vi "SPI Flash Init.vi"(7 "pConfig":T1, 9 "ClockSpeed":i32, 10 "SPIIndex":i32, 11 "DevHandle":i32) -> (3 "function return":i32, 5 "pConfig out":T1)   [LabVIEW 2010, in "usb2spi.lvlib"]
doc: "int WINAPI SPI_FlashInit(int DevHandle,int SPIIndex,int ClockSpeed, PSPI_FLASH_CONFIG pConfig);"
uses:
  usb2spi.lvlib
  USB2XXX/trunk/USB2XXX/USB2XXX/vs2010/Release/USB2XXX.dll
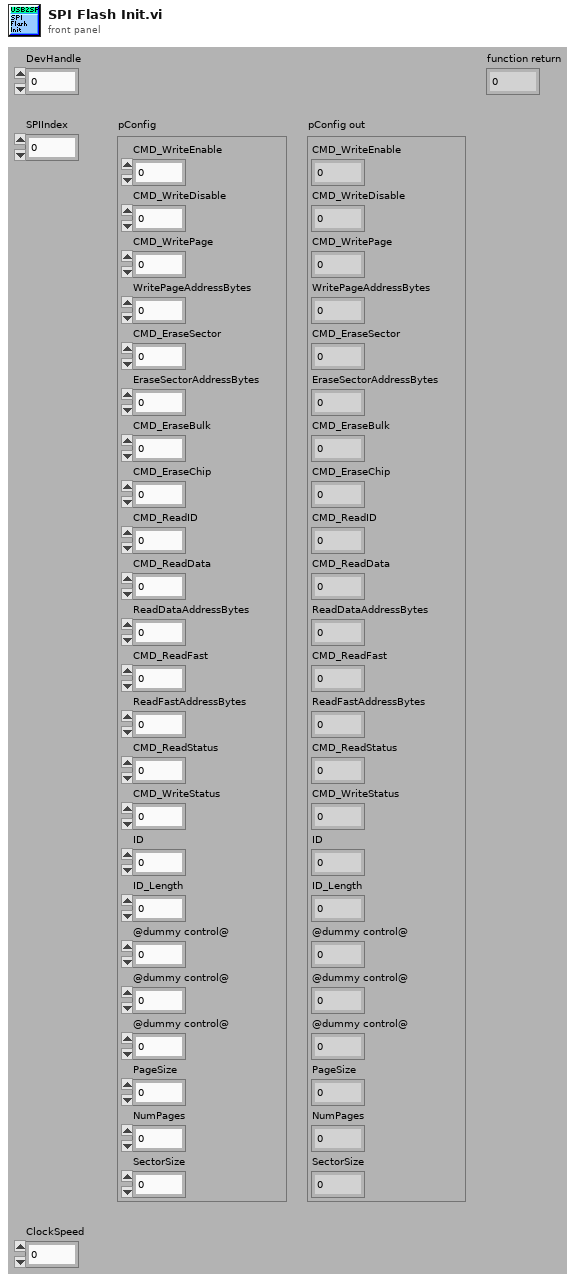
[diagram p1: front panel]
types:
  T1 = cluster{"CMD_WriteEnable":u8, "CMD_WriteDisable":u8, "CMD_WritePage":u8, "WritePageAddressBytes":u8, "CMD_EraseSector":u8, "EraseSectorAddressBytes":u8, "CMD_EraseBulk":u8, "CMD_EraseChip":u8, "CMD_ReadID":u8, "CMD_ReadData":u8, "ReadDataAddressBytes":u8, "CMD_ReadFast":u8, "ReadFastAddressBytes":u8, "CMD_ReadStatus":u8, "CMD_WriteStatus":u8, "ID":u8, "ID_Length":u8, "@dummy control@":i8, "@dummy control@":i8, "@dummy control@":i8, "PageSize":i32, "NumPages":i32, "SectorSize":i32}
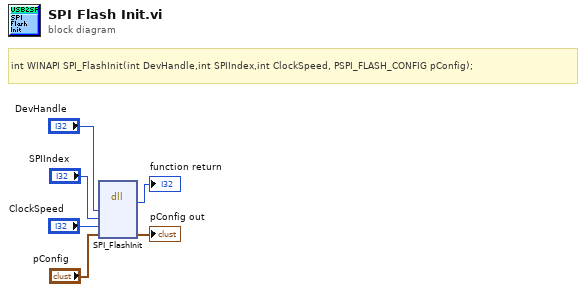
[diagram p0: block diagram]
diagram:
  # "int WINAPI SPI_FlashInit(int DevHandle,int SPIIndex,int ClockSpeed, PSPI_FLASH_CONFIG pConfig);"
  n1 = dll-call lib="E:/OtherWork/STM32/USB2XXX/trunk/USB2XXX/USB2XXX/vs2010/Release/USB2XXX.*" fn="SPI_FlashInit"("DevHandle"="DevHandle", "SPIIndex"="SPIIndex", "ClockSpeed"="ClockSpeed", "pConfig"="pConfig") -> (→"function return":i32, "pConfig"=→"pConfig out":T1)  [unwired: 6 in, 2 out]
